vi "SPIN2_Trim_Meas_ODFT_iHV.vi"(10 "Ext_HV":dbl=38.0 format="%#_13g", 11 "Semiconductor Module Context":T1) -> (0 "error out":errorcluster, 3 "ODFT_Meas":dbl format="%#_6p")   [LabVIEW 2013]
uses:
  <vilib>/NI_TestStand_SemiconductorModule/NI_TestStand_Semiconductor_Module.lvlibp/PinMap/General/SemiconductorModuleContext.ctl
  <instrlib>/niHSDIO/niHSDIO.llb/niHSDIO_ctl Trigger Script - trigID Values (Ring).ctl
  <vilib>/NI_TestStand_SemiconductorModule/NI_TestStand_Semiconductor_Module.lvlibp/PinMap/DC Power/PinsToNIDCPowerSessions.vi
  <vilib>/NI_TestStand_SemiconductorModule/NI_TestStand_Semiconductor_Module.lvlibp
panel:
  in  "Pins":string[](array[string])=["HV"]
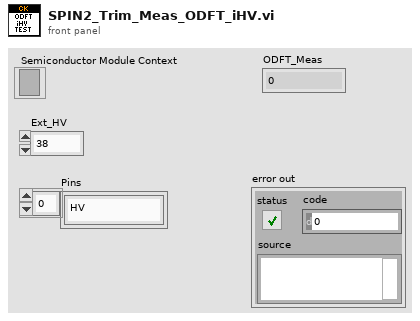
[diagram p1: front panel]
types:
  T1 = typedef "NI_TestStand_Semiconductor_Module.lvlibp/SemiconductorModuleContext.ctl" = refnum<k7>
  T2 = typedef "niHSDIO_ctl Trigger Script - trigID Values (Ring).ctl" = string
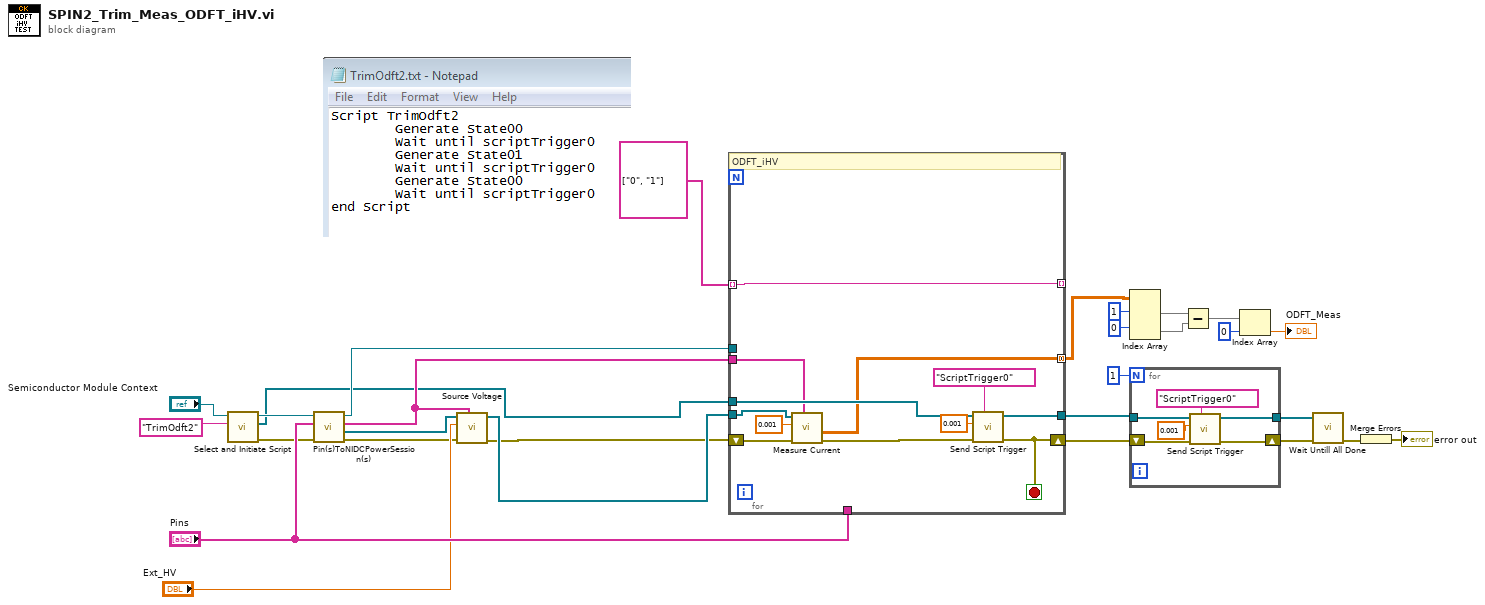
[diagram p0: block diagram]
diagram:
  n1 = call "Select and Initiate Script.vi"("script name"="TrimOdft2", "Semiconductor Module Context"="Semiconductor Module Context") -> ("error out"=w22:errorcluster, "HSDIO GEN Sessions Out"=w2:refnum<k15>[], "Semiconductor Module Context Out"=w23:T1)  [unwired: 7 in]
  n2 = call-poly <vilib>:"Pin(s)ToNIDCPowerSession(s).vi"("error in (no error)"=w22, "Pins"="Pins", "Semiconductor Module Context"=w23) -> ("error out"=w5:errorcluster, "Instrument Sessions"=w4:refnum<k15>[], "Channel Lists"=w21:string[], "Semiconductor Module Context Out"=w25:T1)  [unwired: 4 in, 1 out]
  n3 = call "Source Voltage.vi"("Channel Lists"=w21, "error in (no error)"=w5, "voltage level"="Ext_HV", "Instrument Sessions In"=w4) -> ("error out"=w1:errorcluster, "Instrument Sessions Out"=w3:refnum<k15>[])  [unwired: 4 in, 2 out]
  n4 = for {
    tunnel: string[] ["0", "1"] -> [w41] mode=indexing
    tunnel: w25 -> [_]
    shift-right: [w38] -> w9
    shift-left: w1 -> [w36]
    tunnel: [w41] -> _ mode=indexing
    tunnel: "Pins" -> [_]
    tunnel: w2 -> [w39]
    tunnel: w21 -> [w35]
    tunnel: [w37] -> w16 mode=concatenating
    tunnel: [w34] -> w8
    tunnel: w3 -> [w30]
    stop <- w38 stop-if-true
    # "ODFT_iHV"
    n5 = call "Measure Current.vi"("Channel Lists"=w35, "error in (no error)"=w36, "Delay Time (s)"=0.001, "DCPower Sessions In"=w30) -> ("error out"=w32:errorcluster, "current measurements"=w37:dbl[][])  [unwired: 5 in, 1 out]
    n6 = call "Send Script Trigger.vi"("trigger id (script trigger 0)"=T2 "ScriptTrigger0", "error in (no error)"=w32, "Delay Time (s)"=0.001, "HSDIO Sessions In"=w39) -> ("error out"=w38:errorcluster, "HSDIO Sessions Out"=w34:refnum<k15>[])  [unwired: 6 in]
  }
  n7 = Index Array(array=w16, index (row) #1=1 ("index (row)"), index (row) #2=0 ("index (row)")) -> (element #1=w15:dbl[], element #2=w14:dbl[])  [unwired: 2 in]
  n8 = for {
    N: 1 -> [_]
    shift-right: [w45] -> w7
    shift-left: w9 -> [w46]
    tunnel: w8 -> [w44]
    tunnel: [w43] -> w6
    n9 = call "Send Script Trigger.vi"("trigger id (script trigger 0)"=T2 "ScriptTrigger0", "error in (no error)"=w46, "Delay Time (s)"=0.001, "HSDIO Sessions In"=w44) -> ("error out"=w45:errorcluster, "HSDIO Sessions Out"=w43:refnum<k15>[])  [unwired: 6 in]
  }
  n10 = Subtract(x=w15, y=w14) -> (x-y=w13:dbl[])
  n11 = Index Array(array=w13, index=0) -> (element=→"ODFT_Meas":dbl)
  n12 = call "Wait Untill All Done.vi"("error in (no error)"=w7, "HSDIO Sessions In"=w6) -> ("error out"=w20:errorcluster)  [unwired: 8 in, 1 out]
  n13 = Merge Errors(w20) -> (→"error out":errorcluster)
